vi "Gas-Control-GUI.vi"() -> ()   [LabVIEW 2021]
uses:
  Controls/AR-Auto-Fill.ctl
  Controls/AR-Auto-Purge.ctl
  Controls/AR-DO-Action.ctl
panel:
  out "Data":bool[](array[boolean])
  in  "1000T Sim 2":dbl=1.0
  in  ">750 sim 2":bool=TRUE
  in  "10T Sim 2":dbl=10.0
  in  "<0.1T sim 2":bool
  out "Purge State":T1
  in  "1000T Sim":dbl=1.0
  in  ">750 sim":bool=TRUE
  in  "<0.01T sim":bool
  in  "10T Sim":dbl=10.0
  in  "simulate":bool
  out "Fill State":T2
  out "O2 pwr":bool
  out "Gas SOL":bool
  out "Vac SOL":bool
  in  "Quit":bool
  out "Purge Done":bool
  in  "Auto purge":bool
  out "0-25% O2 (AI2)":dbl caption="0-25% O2" format="%.1f %"
  out "O2 1000ppm (AI3)":dbl caption="1000 PPM O2" format="%.0f PPM"
  out "1000 Torr (AI1)":dbl caption="1000 Torr Gage" format="%.1f Torr"
  out "10 Torr (AI0)":dbl caption="10 Torr Gage" format="%.2f Torr"
  out "Gage Err (DI2)":bool
  out "O2 Timer":dbl format="%.1f sec"
  in  "O2 1000ppm (DO3)":bool
  out "Gas sol timer":dbl caption="Gas Solenoid Timer" format="%.1f sec"
  in  "Gas sol (DO2)":bool
  in  "Vac sol (DO1)":bool
  out "Vac sol timer":dbl caption="Vac Solenoid Timer" format="%.1f sec"
  in  "Pump (DO0)":bool
  out "Fill Done":bool
  in  "Auto fill":bool
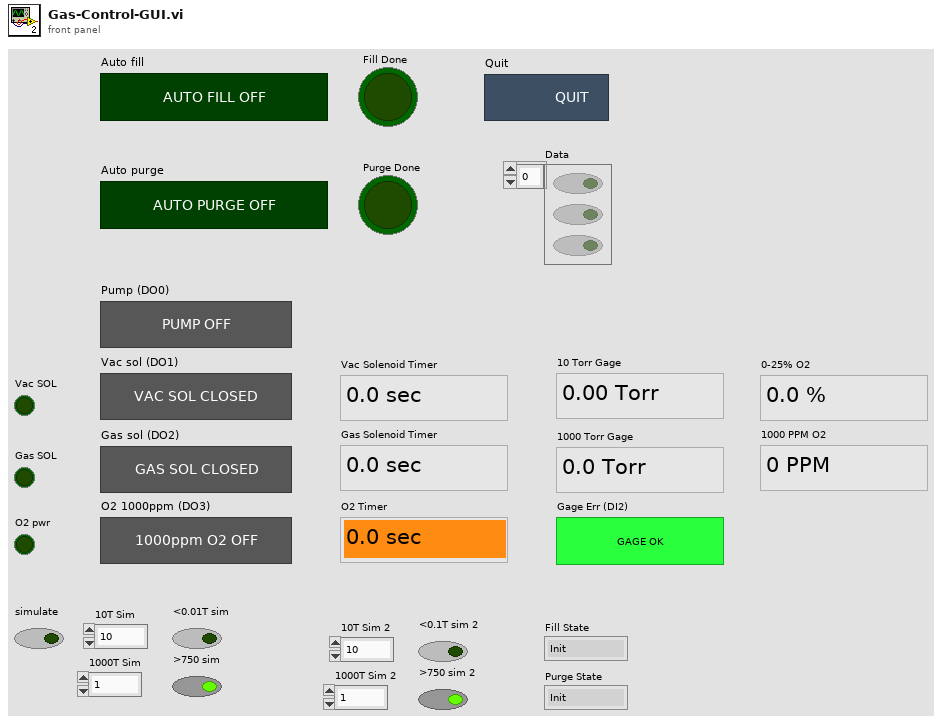
[diagram p1: front panel]
types:
  T1 = typedef "AR-Auto-Purge.ctl" = enum16{"Init", "Start Pump", "Stop Pump", "10T Gage", "1000T Gage", "End"}
  T2 = typedef "AR-Auto-Fill.ctl" = enum16{"Init", "Start Pump", "Stop Pump", "Gas Open", "Gas Close", "10T Gage", "1000T Gage", "End"}
  T3 = typedef "AR-DO-Action.ctl" = enum16{"Init", "Update", "Keep DO3"}
  T4 = enum8{"Enabled", "Disabled", "Disabled and Grayed Out"}
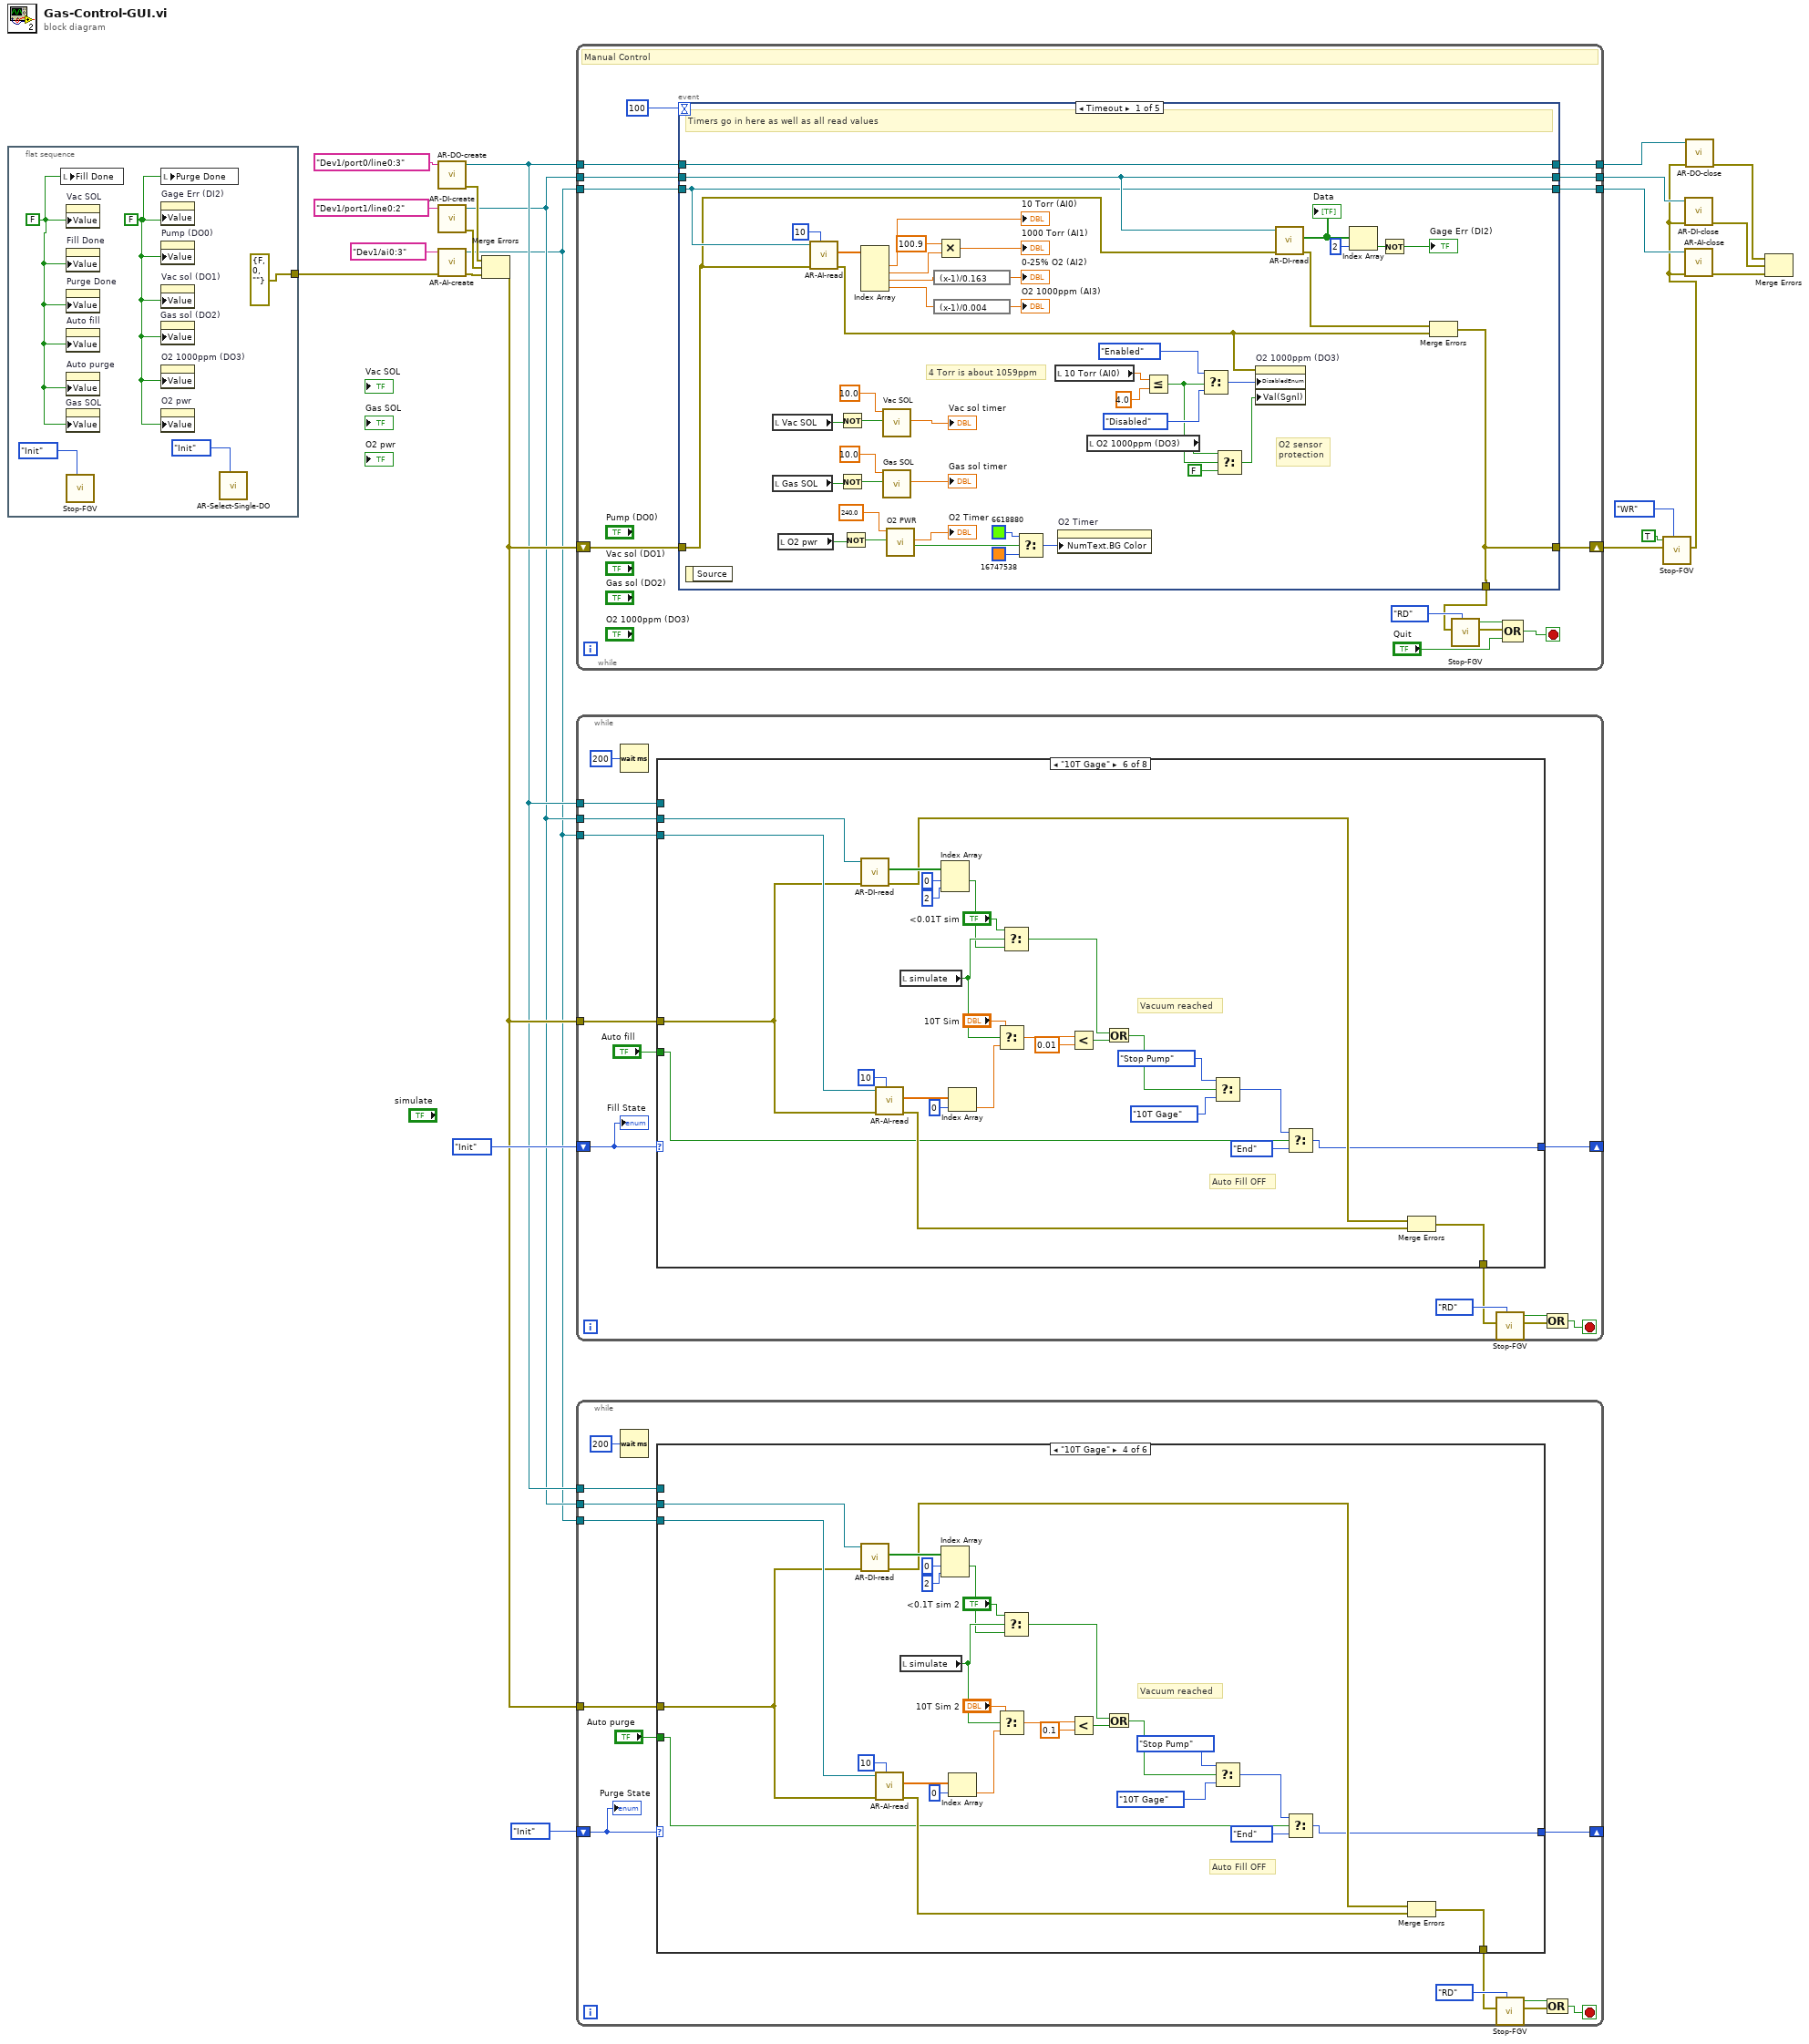
[diagram p0: block diagram]
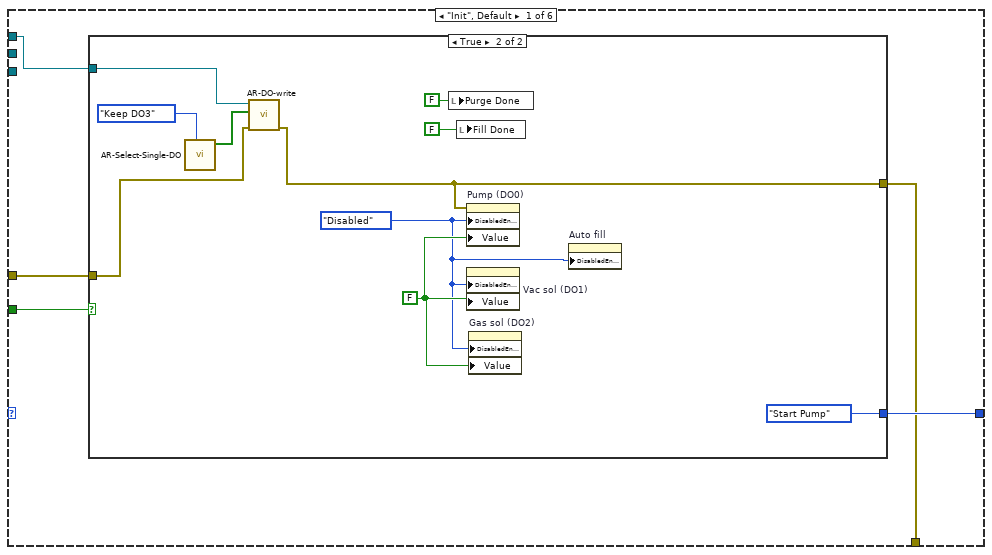
[diagram p2: hidden frame]
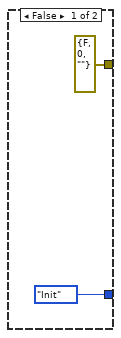
[diagram p3: hidden frame]
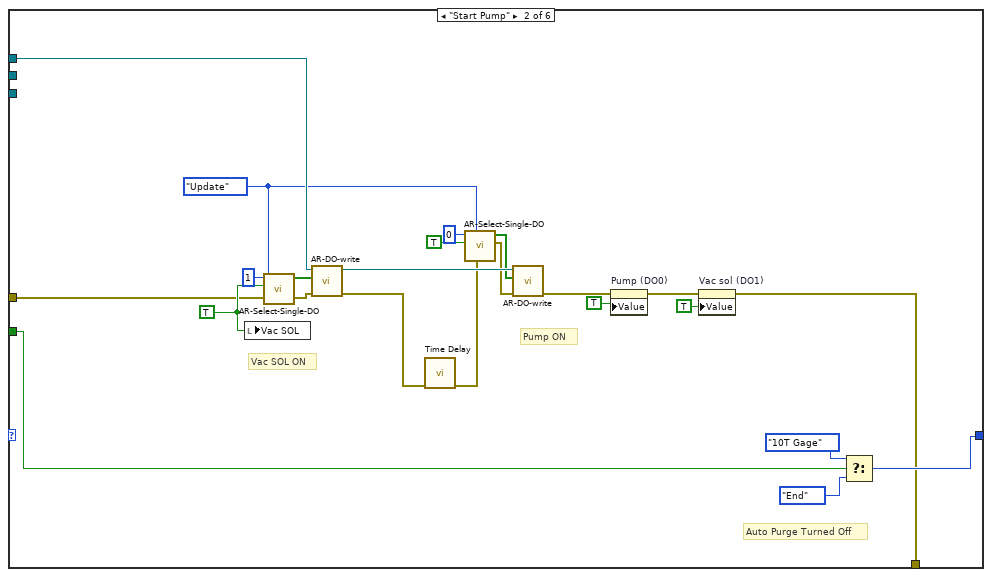
[diagram p4: hidden frame]
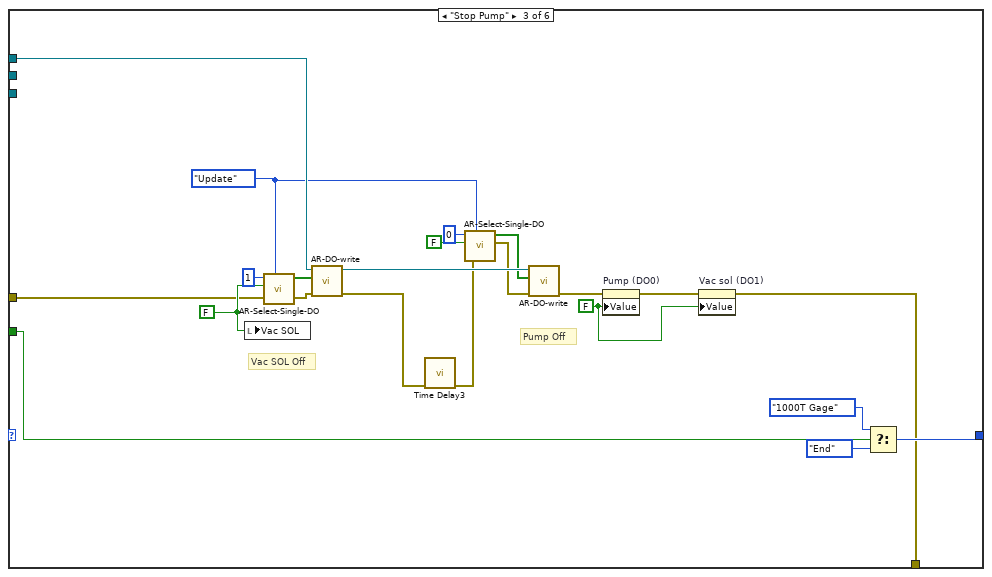
[diagram p5: hidden frame]
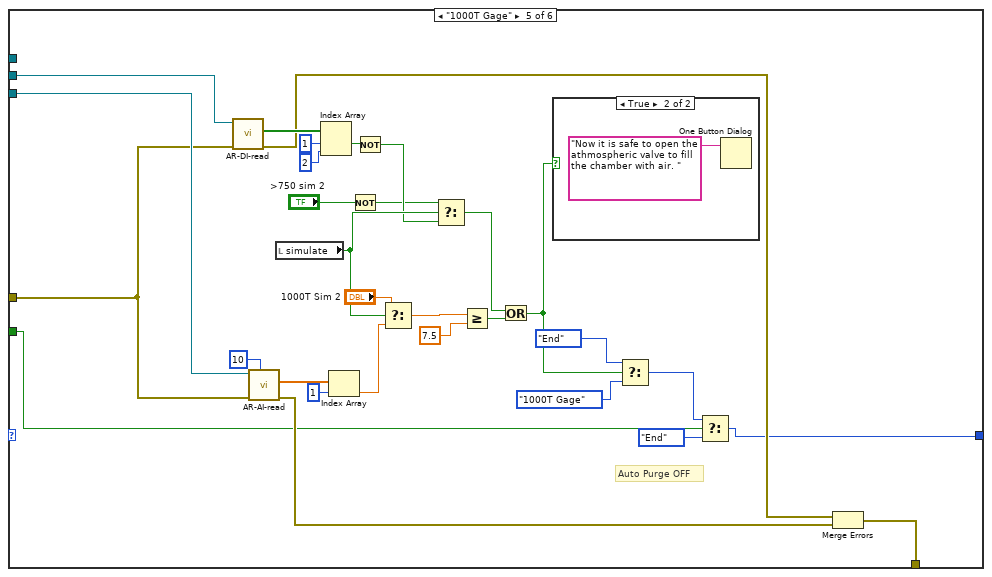
[diagram p6: hidden frame]
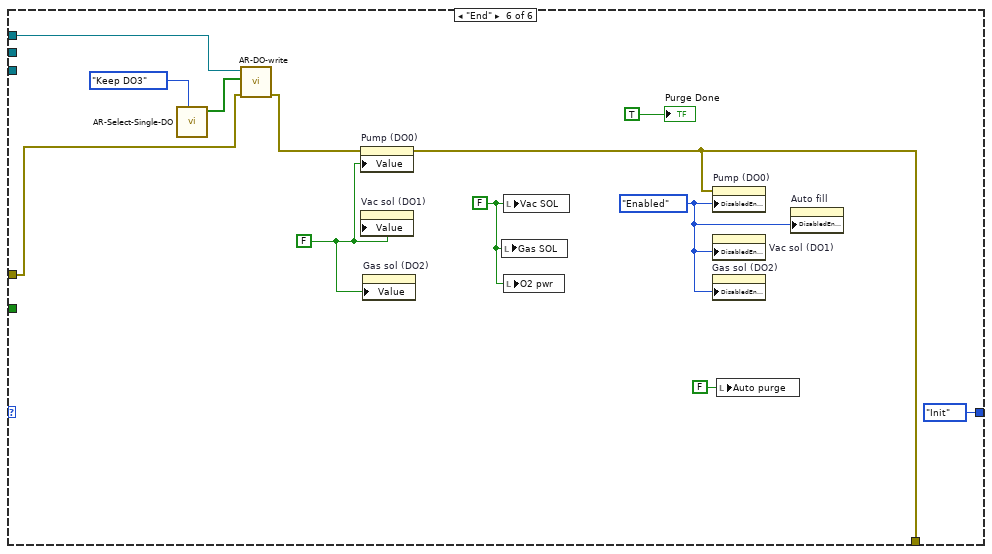
[diagram p8: hidden frame]
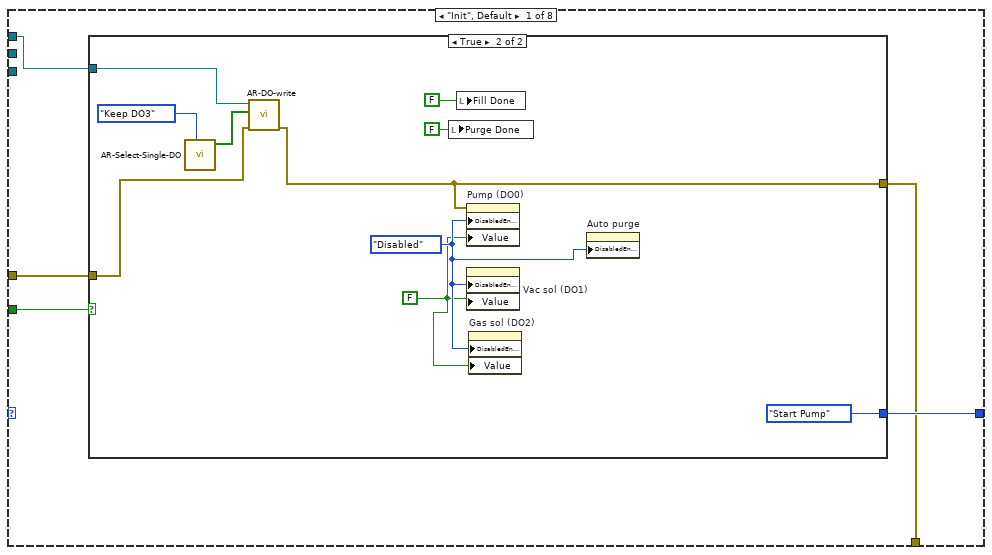
[diagram p9: hidden frame]
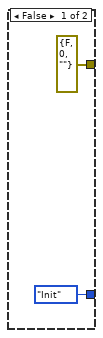
[diagram p10: hidden frame]
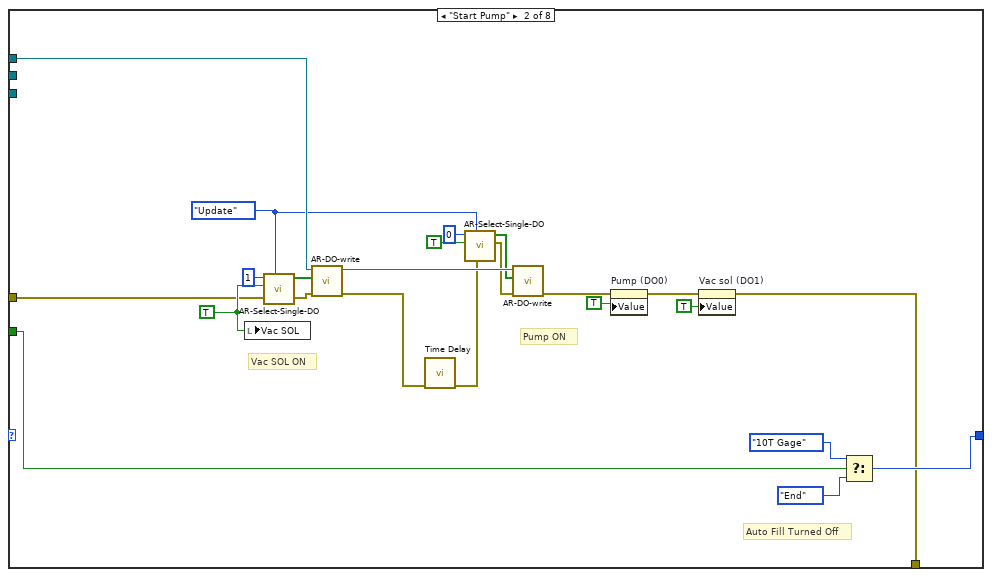
[diagram p11: hidden frame]
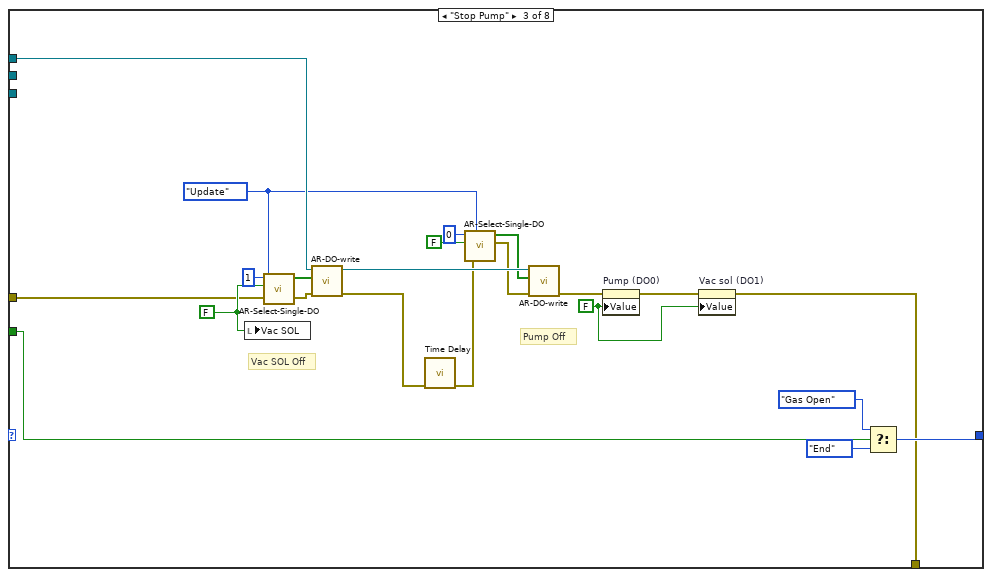
[diagram p12: hidden frame]
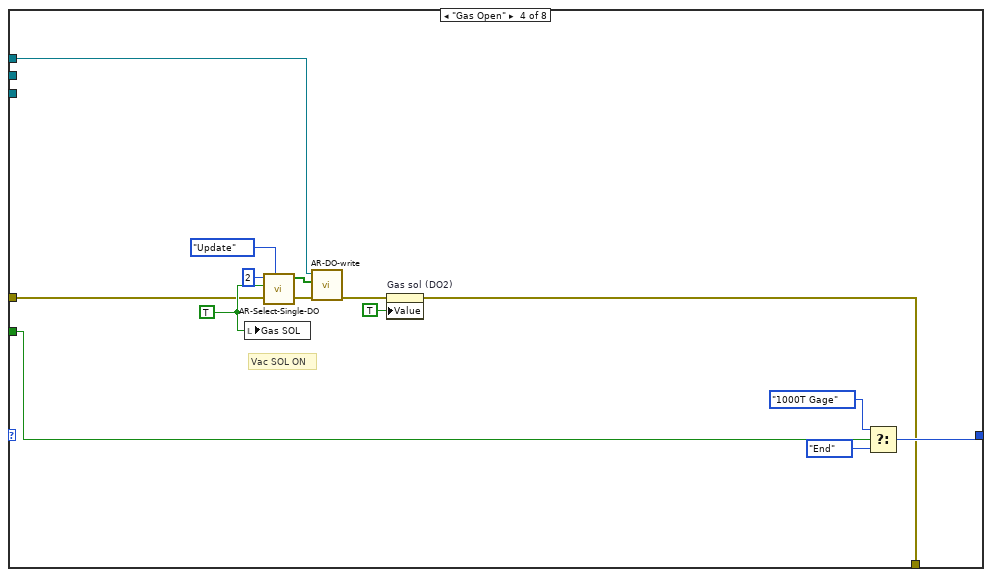
[diagram p13: hidden frame]
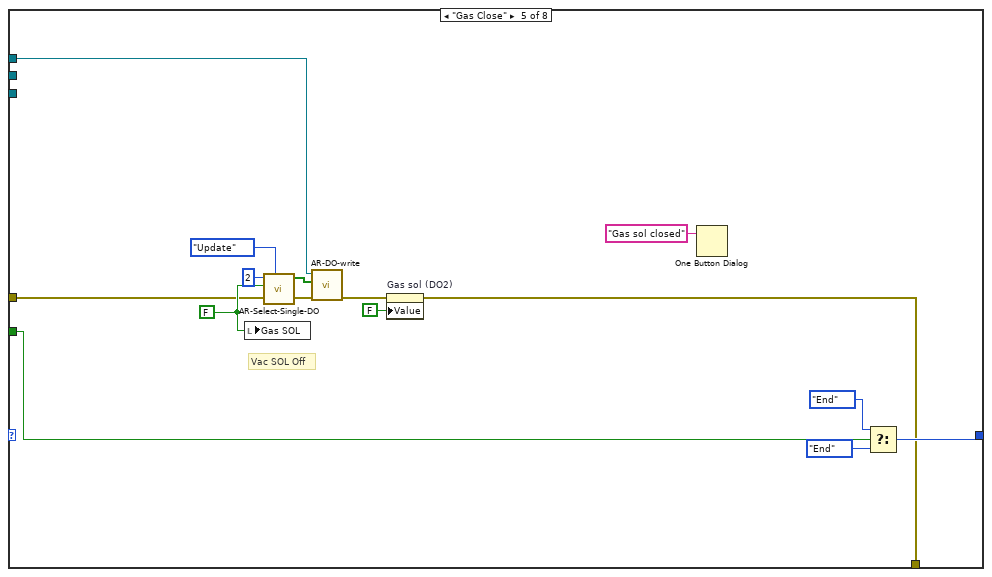
[diagram p14: hidden frame]
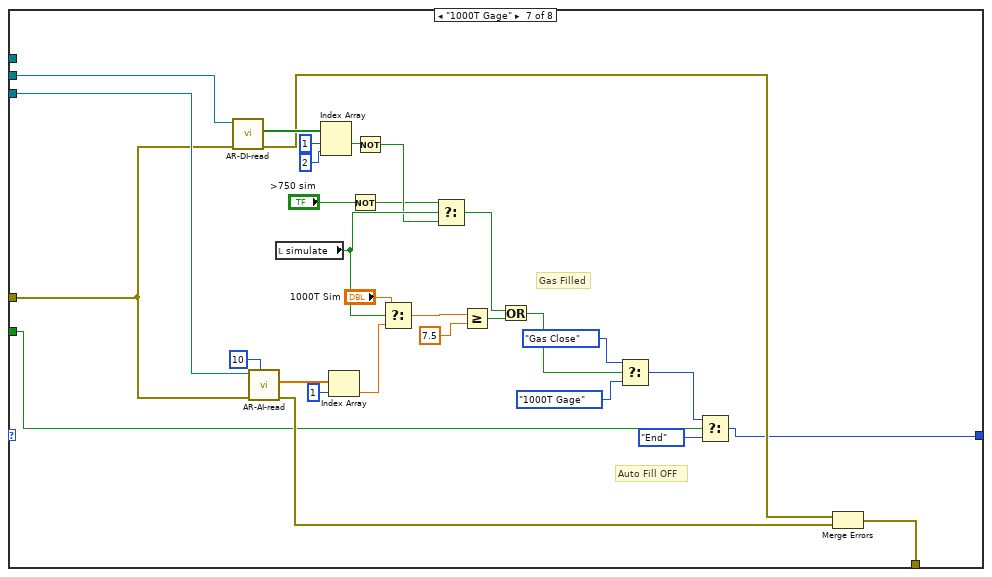
[diagram p15: hidden frame]
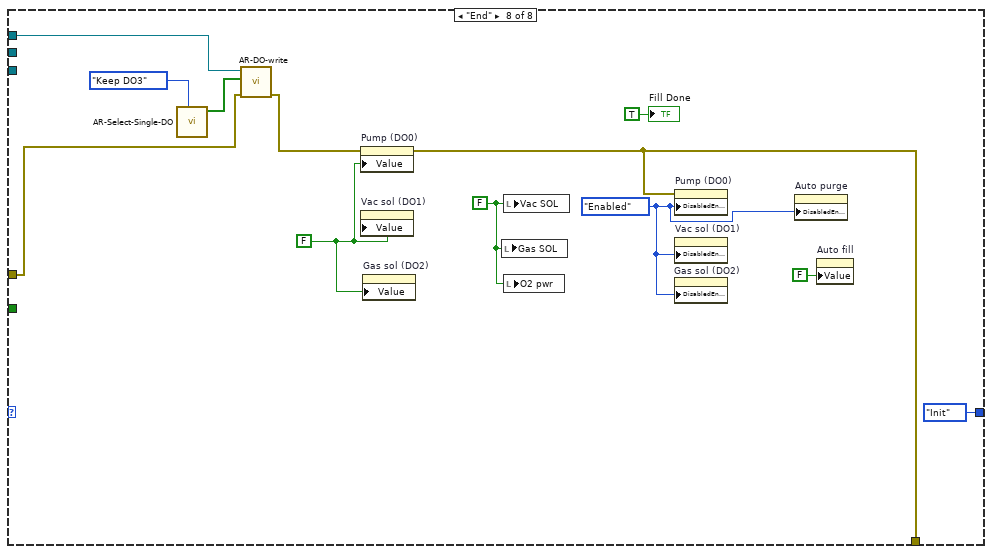
[diagram p16: hidden frame]
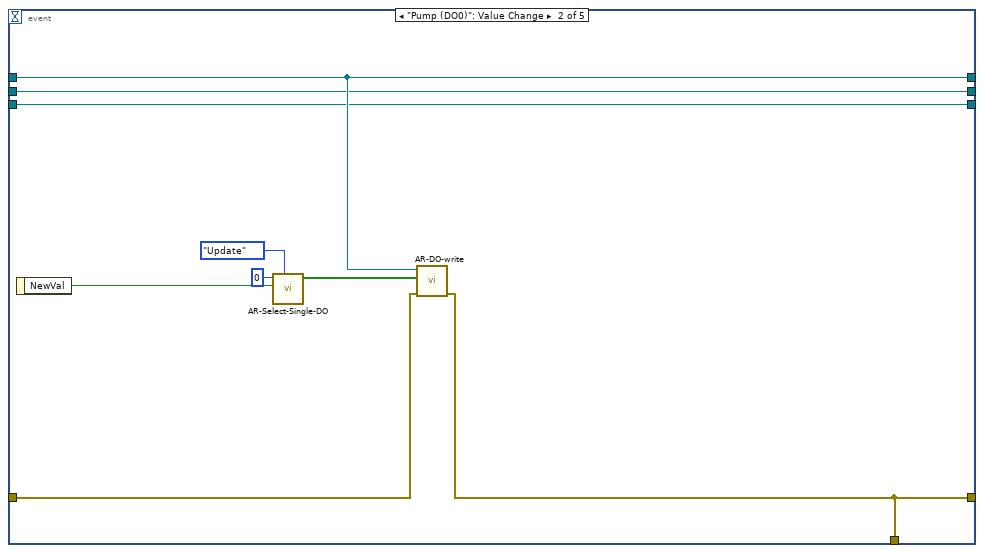
[diagram p17: hidden frame]
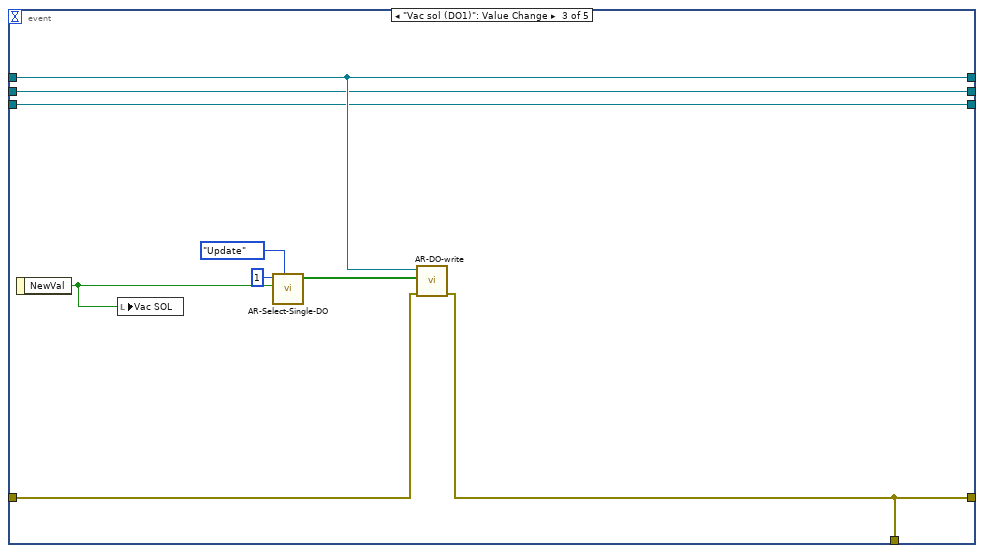
[diagram p18: hidden frame]
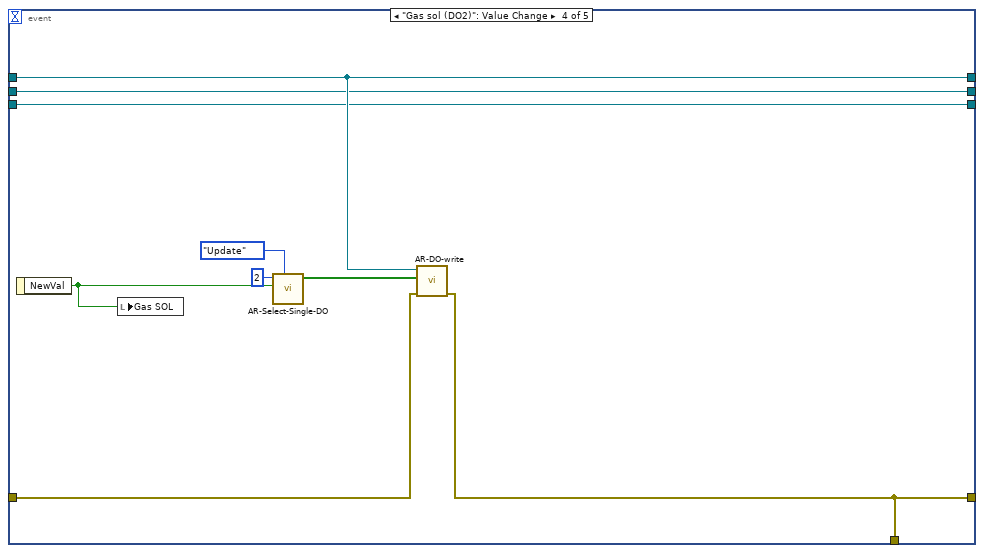
[diagram p19: hidden frame]
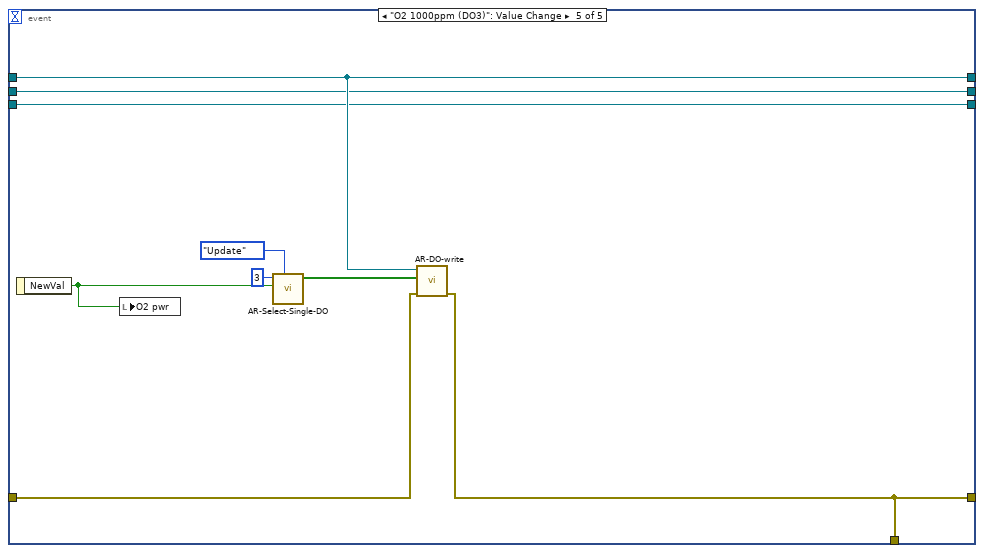
[diagram p20: hidden frame]
diagram:
  n1 = flat-sequence {
    tunnel: [errorcluster {"status"=FALSE, "code"=0, "source"=""} ("error out")] -> w11
    frame #0 {
      w25 = FALSE ("Vac SOL")
      w26 = FALSE ("Vac SOL")
      n2 = local write "Fill Done"(w26) -> ()
      n3 = property on="Vac SOL" class="Bool (strict)"("Value"=w26) -> ()  [unwired: 2 in, 2 out]
      n4 = property on="Fill Done" class="Bool (strict)"("Value"=w26) -> ()  [unwired: 2 in, 2 out]
      n5 = property on="Purge Done" class="Bool (strict)"("Value"=w26) -> ()  [unwired: 2 in, 2 out]
      n6 = property on="Auto fill" class="Bool (strict)"("Value"=w26) -> ()  [unwired: 2 in, 2 out]
      n7 = property on="Auto purge" class="Bool (strict)"("Value"=w26) -> ()  [unwired: 2 in, 2 out]
      n8 = property on="Gas SOL" class="Bool (strict)"("Value"=w26) -> ()  [unwired: 2 in, 2 out]
      n9 = call "Stop-FGV.vi"("Action (RD)"=enum16{"Init", "WR", "RD"}."Init") -> ()  [unwired: 9 in, 2 out]
      n10 = local write "Purge Done"(w25) -> ()
      n11 = property on="Gage Err (DI2)" class="Bool"("Value"=w25) -> ()  [unwired: 2 in, 2 out]
      n12 = property on="Pump (DO0)" class="Bool (strict)"("Value"=w25) -> ()  [unwired: 2 in, 2 out]
      n13 = property on="Vac sol (DO1)" class="Bool (strict)"("Value"=w25) -> ()  [unwired: 2 in, 2 out]
      n14 = property on="Gas sol (DO2)" class="Bool (strict)"("Value"=w25) -> ()  [unwired: 2 in, 2 out]
      n15 = property on="O2 1000ppm (DO3)" class="Bool (strict)"("Value"=w25) -> ()  [unwired: 2 in, 2 out]
      n16 = property on="O2 pwr" class="Bool (strict)"("Value"=w25) -> ()  [unwired: 2 in, 2 out]
      n17 = call "AR-Select-Single-DO.vi"("Action"=AR-DO-Action."Init") -> ()  [unwired: 9 in, 2 out]
    }
  }
  n18 = call "AR-DO-create.vi"("lines"=tag "Dev1/port0/line0:3") -> ("error out"=w14:errorcluster, "DO task out"=w4:refnum<k21>)  [unwired: 9 in]
  n19 = call "AR-DI-create.vi"("lines"=tag "Dev1/port1/line0:2") -> ("error out"=w13:errorcluster, "DI task out"=w3:refnum<k21>)  [unwired: 9 in]
  n20 = call "AR-AI-create.vi"("error in"=w11, "lines"=tag "Dev1/ai0:3") -> ("error out"=w12:errorcluster, "AI task out"=w2:refnum<k21>)  [unwired: 8 in]
  n21 = Merge Errors(w14, w13, w12) -> (w5:errorcluster)
  n22 = while {
    tunnel: w4 -> [w42]
    tunnel: w3 -> [w41]
    tunnel: w2 -> [w40]
    shift-right: [w39] -> w8
    shift-left: w5 -> [w38]
    tunnel: [w35] -> w20
    tunnel: [w34] -> w19
    tunnel: [w33] -> w18
    stop <- w37 stop-if-true
    # "Manual Control"
    n23 = event shown="[0] Timeout" {
      selector: _ -> [_ _ _ _ _]
      dyn-events: _ -> [_ _ _ _ _]
      timeout: 100 -> [_ _ _ _ _]
      tunnel: w42 -> [w80 w92 w102 w111 w120]
      tunnel: w41 -> [w79 w91 w101 w110 w119]
      tunnel: w40 -> [w78 w90 w100 w109 w118]
      tunnel: [w77 w93 w103 w112 w121] -> w39
      tunnel: w38 -> [w75 w94 w104 w113 w122]
      tunnel: [w77 w93 w103 w112 w121] -> w31
      tunnel: [w80 w92 w102 w111 w120] -> w35
      tunnel: [w79 w91 w101 w110 w119] -> w34
      tunnel: [w78 w90 w100 w109 w118] -> w33
      event Timeout {
        # "O2 sensor\nprotection"
        # "4 Torr is about 1059ppm"
        # "Timers go in here as well as all read values"
        n24 = event-data() -> ()  [unwired: 1 in, 1 out]
        n25 = local read "Vac SOL"() -> (w88:bool)
        n26 = local read "Gas SOL"() -> (w73:bool)
        n27 = local read "O2 pwr"() -> (w69:bool)
        n28 = call "AR-AI-read.vi"("number of samples"=10, "error in"=w75, "AI task in"=w78) -> ("error out"=w51:errorcluster, "Data"=w83:dbl[])  [unwired: 6 in, 1 out]
        n29 = Not(x=w88) -> (.not. x?=w89:bool)
        n30 = Not(x=w73) -> (.not. x?=w72:bool)
        n31 = Not(x=w69) -> (.not. x?=w70:bool)
        n32 = Index Array(array=w83) -> (element #1=→"10 Torr (AI0)":dbl, element #2=w62:dbl, element #3=w59:dbl, element #4=w56:dbl)  [unwired: 4 in]
        n33 = call "Vac SOL"("Time Target (s)"=10.0, "Reset"=w89) -> ("Elapsed Time (s)"=→"Vac sol timer":dbl)  [unwired: 10 in, 7 out]
        n34 = call "Gas SOL"("Time Target (s)"=10.0, "Reset"=w72) -> ("Elapsed Time (s)"=→"Gas sol timer":dbl)  [unwired: 10 in, 7 out]
        n35 = call "O2 PWR"("Time Target (s)"=240.0, "Reset"=w70) -> ("Elapsed Time (s)"=→"O2 Timer":dbl, "Time has Elapsed"=w65:bool)  [unwired: 10 in, 6 out]
        n36 = expression code="(x-1)/0.163"(w59) -> (→"0-25% O2 (AI2)":dbl)
        n37 = expression code="(x-1)/0.004"(w56) -> (→"O2 1000ppm (AI3)":dbl)
        n38 = Multiply(x=100.9, y=w62) -> (x*y=→"1000 Torr (AI1)":dbl)
        n39 = Select(t=u32 6618880 ("Numeric Text.Colors:BG Color"), s=w65, f=u32 16747538 ("Numeric Text.Colors:BG Color")) -> (s? t:f=w63:u32)
        n40 = local read "10 Torr (AI0)"() -> (w55:dbl)
        n41 = property on="O2 Timer" class="DigNum (strict)"("NumText.BG Color"=w63) -> ()  [unwired: 2 in, 2 out]
        n42 = local read "O2 1000ppm (DO3)"() -> (w48:bool)
        n43 = Less Or Equal?(x=w55, y=4.0) -> (x <= y?=w49:bool)
        n44 = Select(t=T4."Enabled" ("Disabled"), s=w49, f=T4."Disabled" ("Disabled")) -> (s? t:f=w50:T4)
        n45 = Select(t=w48, s=w49, f=FALSE) -> (s? t:f=w46:bool)
        n46 = property on="O2 1000ppm (DO3)" class="Bool (strict)"(error in=w51, "DisabledEnum"=w50, "Val(Sgnl)"=w46) -> ()  [unwired: 1 in, 2 out]
        n47 = call "AR-DI-read.vi"("error in"=w75, "DI task in"=w79) -> ("error out"=w81:errorcluster, "Data"=w86:bool[])  [unwired: 7 in, 1 out]
        "Data" <- w86
        n48 = Index Array(array=w86, index=2) -> (element=w45:bool)
        n49 = Not(x=w45) -> (.not. x?=→"Gage Err (DI2)":bool)
        n50 = Merge Errors(w81, w51) -> (w77:errorcluster)
      }
      event "Pump (DO0)": Value Change {
        n51 = event-data() -> ("NewVal"=w95:bool)  [unwired: 1 in]
        n52 = call "AR-Select-Single-DO.vi"("Action"=enum16{"Init", "Update"}."Update", "DO"=w95, "index"=0) -> ("DO Data"=w97:bool[])  [unwired: 7 in, 1 out]
        n53 = call "AR-DO-write.vi"("error in (no error)"=w94, "Data"=w97, "DO task in"=w92) -> ("error out"=w93:errorcluster)  [unwired: 7 in, 1 out]
      }
      event "Vac sol (DO1)": Value Change {
        n54 = event-data() -> ("NewVal"=w99:bool)  [unwired: 1 in]
        n55 = local write "Vac SOL"(w99) -> ()
        n56 = call "AR-Select-Single-DO.vi"("Action"=enum16{"Init", "Update"}."Update", "DO"=w99, "index"=1) -> ("DO Data"=w106:bool[])  [unwired: 7 in, 1 out]
        n57 = call "AR-DO-write.vi"("error in (no error)"=w104, "Data"=w106, "DO task in"=w102) -> ("error out"=w103:errorcluster)  [unwired: 7 in, 1 out]
      }
      event "Gas sol (DO2)": Value Change {
        n58 = event-data() -> ("NewVal"=w108:bool)  [unwired: 1 in]
        n59 = local write "Gas SOL"(w108) -> ()
        n60 = call "AR-Select-Single-DO.vi"("Action"=enum16{"Init", "Update"}."Update", "DO"=w108, "index"=2) -> ("DO Data"=w115:bool[])  [unwired: 7 in, 1 out]
        n61 = call "AR-DO-write.vi"("error in (no error)"=w113, "Data"=w115, "DO task in"=w111) -> ("error out"=w112:errorcluster)  [unwired: 7 in, 1 out]
      }
      event "O2 1000ppm (DO3)": Value Change {
        n62 = event-data() -> ("NewVal"=w117:bool)  [unwired: 1 in]
        n63 = local write "O2 pwr"(w117) -> ()
        n64 = call "AR-Select-Single-DO.vi"("Action"=enum16{"Init", "Update"}."Update", "DO"=w117, "index"=3) -> ("DO Data"=w124:bool[])  [unwired: 7 in, 1 out]
        n65 = call "AR-DO-write.vi"("error in (no error)"=w122, "Data"=w124, "DO task in"=w120) -> ("error out"=w121:errorcluster)  [unwired: 7 in, 1 out]
      }
    }
    n66 = call "Stop-FGV.vi"("Action (RD)"=enum16{"Init", "WR", "RD"}."RD", "error in"=w31) -> ("error out"=w30:errorcluster, "Out"=w29:bool)  [unwired: 8 in]
    n67 = Compound Arithmetic op=OR(w29, w30, "Quit") -> (w37:bool)
  }
  n68 = while {
    tunnel: w4 -> [w130]
    tunnel: w3 -> [w126]
    tunnel: w2 -> [w127]
    shift-right: [w132] -> _
    shift-left: AR-Auto-Fill."Init" ("Fill State") -> [w131]
    tunnel: w5 -> [w128]
    stop <- w135 stop-if-true
    n69 = Wait (ms)(milliseconds to wait=u32 200) -> ()  [unwired: 1 out]
    n70 = case shown="\"10T Gage\"" w131 {
      tunnel: "Auto fill" -> [w143 w167 w188 w206 w220 w230 w262 _]
      tunnel: [w142 w164 w185 w203 w217 w227 w259 AR-Auto-Fill."Init" ("f")] -> w132
      tunnel: w130 -> [w141 w175 w196 w209 w223 _ _ w292]
      tunnel: [w140 w159 w181 w201 w215 w231 w263 w285] -> w129
      tunnel: w128 -> [w139 w168 w189 w207 w221 w244 w274 w291]
      tunnel: w127 -> [_ _ _ _ _ w252 w282 _]
      tunnel: w126 -> [_ _ _ _ _ w245 w275 _]
      frame "Init", Default {
        n71 = case shown="True" w143 {
          tunnel: [AR-Auto-Fill."Init" ("Fill State") AR-Auto-Fill."Start Pump" ("Fill State")] -> w142
          tunnel: w141 -> [_ w153]
          tunnel: [errorcluster {"status"=FALSE, "code"=0, "source"=""} ("error out") w149] -> w140
          tunnel: w139 -> [_ w151]
          frame False {
          }
          frame True {
            w150 = FALSE
            w155 = T4."Disabled" ("Disabled")
            n72 = call "AR-Select-Single-DO.vi"("Action"=AR-DO-Action."Keep DO3") -> ("DO Data"=w152:bool[])  [unwired: 9 in, 1 out]
            n73 = call "AR-DO-write.vi"("error in (no error)"=w151, "Data"=w152, "DO task in"=w153) -> ("error out"=w149:errorcluster)  [unwired: 7 in, 1 out]
            n74 = local write "Purge Done"(FALSE ("Purge Done")) -> ()
            n75 = local write "Fill Done"(FALSE ("Purge Done")) -> ()
            n76 = property on="Pump (DO0)" class="Bool (strict)"(error in=w149, "DisabledEnum"=w155, "Value"=w150) -> ()  [unwired: 1 in, 2 out]
            n77 = property on="Vac sol (DO1)" class="Bool (strict)"("DisabledEnum"=w155, "Value"=w150) -> ()  [unwired: 2 in, 2 out]
            n78 = property on="Gas sol (DO2)" class="Bool (strict)"("DisabledEnum"=w155, "Value"=w150) -> ()  [unwired: 2 in, 2 out]
            n79 = property on="Auto purge" class="Bool (strict)"("DisabledEnum"=w155) -> ()  [unwired: 2 in, 2 out]
          }
        }
      }
      frame "Start Pump" {
        w156 = AR-DO-Action."Update" ("Action")
        w174 = TRUE ("DO")
        # "Auto Fill Turned Off"
        # "Pump ON"
        # "Vac SOL ON"
        n80 = local write "Vac SOL"(w174) -> ()
        n81 = call "AR-Select-Single-DO.vi"("Action"=w156, "DO"=w174, "index"=1) -> ("DO Data"=w176:bool[])  [unwired: 7 in, 1 out]
        n82 = call "AR-DO-write.vi"("error in (no error)"=w168, "Data"=w176, "DO task in"=w175) -> ("error out"=w169:errorcluster, "DO task out"=w172:refnum<k21>)  [unwired: 7 in]
        n83 = call "Time Delay"("error in (no error)"=w169) -> ("error out"=w158:errorcluster)  [unwired: 10 in]
        n84 = call "AR-Select-Single-DO.vi"("error in (no error)"=w158, "Action"=w156, "DO"=TRUE, "index"=0) -> ("error out"=w157:errorcluster, "DO Data"=w171:bool[])  [unwired: 6 in]
        n85 = call "AR-DO-write.vi"("error in (no error)"=w157, "Data"=w171, "DO task in"=w172) -> ("error out"=w162:errorcluster)  [unwired: 7 in, 1 out]
        n86 = property on="Pump (DO0)" class="Bool (strict)"(error in=w162, "Value"=TRUE ("Pump (DO0)")) -> (error out=w161:errorcluster)  [unwired: 1 in, 1 out]
        n87 = property on="Vac sol (DO1)" class="Bool (strict)"(error in=w161, "Value"=TRUE ("Vac sol (DO1)")) -> (error out=w159:errorcluster)  [unwired: 1 in, 1 out]
        n88 = Select(t=AR-Auto-Fill."10T Gage" ("Fill State"), s=w167, f=AR-Auto-Fill."End" ("Fill State")) -> (s? t:f=w164:T2)
      }
      frame "Stop Pump" {
        w178 = AR-DO-Action."Update" ("Action")
        w182 = FALSE ("Pump (DO0)")
        w195 = FALSE ("DO")
        # "Pump Off"
        # "Vac SOL Off"
        n89 = local write "Vac SOL"(w195) -> ()
        n90 = call "AR-Select-Single-DO.vi"("Action"=w178, "DO"=w195, "index"=1) -> ("DO Data"=w197:bool[])  [unwired: 7 in, 1 out]
        n91 = call "AR-DO-write.vi"("error in (no error)"=w189, "Data"=w197, "DO task in"=w196) -> ("error out"=w190:errorcluster, "DO task out"=w193:refnum<k21>)  [unwired: 7 in]
        n92 = call "Time Delay"("error in (no error)"=w190) -> ("error out"=w180:errorcluster)  [unwired: 10 in]
        n93 = call "AR-Select-Single-DO.vi"("error in (no error)"=w180, "Action"=w178, "DO"=FALSE, "index"=0) -> ("error out"=w179:errorcluster, "DO Data"=w192:bool[])  [unwired: 6 in]
        n94 = call "AR-DO-write.vi"("error in (no error)"=w179, "Data"=w192, "DO task in"=w193) -> ("error out"=w184:errorcluster)  [unwired: 7 in, 1 out]
        n95 = property on="Pump (DO0)" class="Bool (strict)"(error in=w184, "Value"=w182) -> (error out=w183:errorcluster)  [unwired: 1 in, 1 out]
        n96 = property on="Vac sol (DO1)" class="Bool (strict)"(error in=w183, "Value"=w182) -> (error out=w181:errorcluster)  [unwired: 1 in, 1 out]
        n97 = Select(t=AR-Auto-Fill."Gas Open" ("Fill State"), s=w188, f=AR-Auto-Fill."End") -> (s? t:f=w185:T2)
      }
      frame "Gas Open" {
        w208 = TRUE ("DO")
        # "Vac SOL ON"
        n98 = local write "Gas SOL"(w208) -> ()
        n99 = call "AR-Select-Single-DO.vi"("Action"=AR-DO-Action."Update", "DO"=w208, "index"=2) -> ("DO Data"=w210:bool[])  [unwired: 7 in, 1 out]
        n100 = call "AR-DO-write.vi"("error in (no error)"=w207, "Data"=w210, "DO task in"=w209) -> ("error out"=w202:errorcluster)  [unwired: 7 in, 1 out]
        n101 = property on="Gas sol (DO2)" class="Bool (strict)"(error in=w202, "Value"=TRUE ("Gas sol (DO2)")) -> (error out=w201:errorcluster)  [unwired: 1 in, 1 out]
        n102 = Select(t=AR-Auto-Fill."1000T Gage" ("Fill State"), s=w206, f=AR-Auto-Fill."End") -> (s? t:f=w203:T2)
      }
      frame "Gas Close" {
        w222 = FALSE ("DO")
        # "Vac SOL Off"
        n103 = local write "Gas SOL"(w222) -> ()
        n104 = call "AR-Select-Single-DO.vi"("Action"=AR-DO-Action."Update", "DO"=w222, "index"=2) -> ("DO Data"=w224:bool[])  [unwired: 7 in, 1 out]
        n105 = call "AR-DO-write.vi"("error in (no error)"=w221, "Data"=w224, "DO task in"=w223) -> ("error out"=w216:errorcluster)  [unwired: 7 in, 1 out]
        n106 = property on="Gas sol (DO2)" class="Bool (strict)"(error in=w216, "Value"=FALSE ("Gas sol (DO2)")) -> (error out=w215:errorcluster)  [unwired: 1 in, 1 out]
        n107 = One Button Dialog(message="Gas sol closed") -> ()  [unwired: 1 in, 1 out]
        n108 = Select(t=AR-Auto-Fill."End" ("Fill State"), s=w220, f=AR-Auto-Fill."End") -> (s? t:f=w217:T2)
      }
      frame "10T Gage" {
        # "Auto Fill OFF"
        # "Vacuum reached"
        n109 = call "AR-DI-read.vi"("error in"=w244, "DI task in"=w245) -> ("error out"=w232:errorcluster, "Data"=w243:bool[])  [unwired: 7 in, 1 out]
        n110 = call "AR-AI-read.vi"("number of samples"=10, "error in"=w244, "AI task in"=w252) -> ("error out"=w233:errorcluster, "Data"=w251:dbl[])  [unwired: 6 in, 1 out]
        n111 = local read "simulate"() -> (w240:bool)
        n112 = Index Array(array=w243, index #1=0 ("index"), index #2=2 ("index")) -> (element #1=w239:bool)  [unwired: 1 out]
        n113 = Index Array(array=w251, index=0) -> (element=w249:dbl)
        n114 = Select(t="10T Sim", s=w240, f=w249) -> (s? t:f=w247:dbl)
        n115 = Select(t="<0.01T sim", s=w240, f=w239) -> (s? t:f=w237:bool)
        n116 = Less?(x=w247, y=0.01) -> (x < y?=w226:bool)
        n117 = Or(x=w237, y=w226) -> (x .or. y?=w236:bool)
        n118 = Select(t=AR-Auto-Fill."Stop Pump" ("Fill State"), s=w236, f=AR-Auto-Fill."10T Gage") -> (s? t:f=w229:T2)
        n119 = Select(t=w229, s=w230, f=AR-Auto-Fill."End") -> (s? t:f=w227:T2)
        n120 = Merge Errors(w232, w233) -> (w231:errorcluster)
      }
      frame "1000T Gage" {
        # "Auto Fill OFF"
        # "Gas Filled"
        n121 = call "AR-DI-read.vi"("error in"=w274, "DI task in"=w275) -> ("error out"=w264:errorcluster, "Data"=w273:bool[])  [unwired: 7 in, 1 out]
        n122 = call "AR-AI-read.vi"("number of samples"=10, "error in"=w274, "AI task in"=w282) -> ("error out"=w265:errorcluster, "Data"=w281:dbl[])  [unwired: 6 in, 1 out]
        n123 = local read "simulate"() -> (w270:bool)
        n124 = Index Array(array=w273, index #1=1 ("index"), index #2=2 ("index")) -> (element #1=w258:bool)  [unwired: 1 out]
        n125 = Index Array(array=w281, index=1) -> (element=w279:dbl)
        n126 = Not(x=">750 sim") -> (.not. x?=w255:bool)
        n127 = Not(x=w258) -> (.not. x?=w257:bool)
        n128 = Select(t="1000T Sim", s=w270, f=w279) -> (s? t:f=w277:dbl)
        n129 = Select(t=w255, s=w270, f=w257) -> (s? t:f=w269:bool)
        n130 = Greater Or Equal?(x=w277, y=7.5) -> (x >= y?=w254:bool)
        n131 = Or(x=w269, y=w254) -> (x .or. y?=w268:bool)
        n132 = Select(t=AR-Auto-Fill."Gas Close" ("Fill State"), s=w268, f=AR-Auto-Fill."1000T Gage") -> (s? t:f=w261:T2)
        n133 = Select(t=w261, s=w262, f=AR-Auto-Fill."End") -> (s? t:f=w259:T2)
        n134 = Merge Errors(w264, w265) -> (w263:errorcluster)
      }
      frame "End" {
        w286 = T4."Enabled" ("Disabled")
        w288 = FALSE ("Vac SOL")
        w289 = FALSE
        n135 = call "AR-Select-Single-DO.vi"("Action"=AR-DO-Action."Keep DO3") -> ("DO Data"=w293:bool[])  [unwired: 9 in, 1 out]
        n136 = call "AR-DO-write.vi"("error in (no error)"=w291, "Data"=w293, "DO task in"=w292) -> ("error out"=w290:errorcluster)  [unwired: 7 in, 1 out]
        n137 = property on="Pump (DO0)" class="Bool (strict)"(error in=w290, "Value"=w289) -> (error out=w285:errorcluster)  [unwired: 1 in, 1 out]
        n138 = property on="Vac sol (DO1)" class="Bool (strict)"("Value"=w289) -> ()  [unwired: 2 in, 2 out]
        n139 = property on="Gas sol (DO2)" class="Bool (strict)"("Value"=w289) -> ()  [unwired: 2 in, 2 out]
        n140 = local write "Gas SOL"(w288) -> ()
        n141 = local write "Vac SOL"(w288) -> ()
        n142 = local write "O2 pwr"(w288) -> ()
        n143 = property on="Pump (DO0)" class="Bool (strict)"(error in=w285, "DisabledEnum"=w286) -> ()  [unwired: 1 in, 2 out]
        n144 = property on="Vac sol (DO1)" class="Bool (strict)"("DisabledEnum"=w286) -> ()  [unwired: 2 in, 2 out]
        n145 = property on="Gas sol (DO2)" class="Bool (strict)"("DisabledEnum"=w286) -> ()  [unwired: 2 in, 2 out]
        n146 = property on="Auto purge" class="Bool (strict)"("DisabledEnum"=w286) -> ()  [unwired: 2 in, 2 out]
        n147 = property on="Auto fill" class="Bool (strict)"("Value"=FALSE ("Auto fill")) -> ()  [unwired: 2 in, 2 out]
        "Fill Done" <- TRUE ("Fill Done")
      }
    }
    n148 = call "Stop-FGV.vi"("Action (RD)"=enum16{"Init", "WR", "RD"}."RD", "error in"=w129) -> ("error out"=w137:errorcluster, "Out"=w138:bool)  [unwired: 8 in]
    n149 = Compound Arithmetic op=OR(w138, w137) -> (w135:bool)
    "Fill State" <- w131
  }
  n150 = while {
    tunnel: w4 -> [w301]
    tunnel: w3 -> [w297]
    tunnel: w2 -> [w298]
    shift-right: [w303] -> _
    shift-left: AR-Auto-Purge."Init" ("Purge State") -> [w302]
    tunnel: w5 -> [w299]
    stop <- w305 stop-if-true
    n151 = Wait (ms)(milliseconds to wait=u32 200) -> ()  [unwired: 1 out]
    n152 = case shown="\"10T Gage\"" w302 {
      tunnel: "Auto purge" -> [w313 w337 w358 w373 w406 _]
      tunnel: [w312 w334 w355 w370 w403 AR-Auto-Purge."Init" ("f")] -> w303
      tunnel: w301 -> [w311 w345 w366 _ _ w437]
      tunnel: [w310 w329 w351 w374 w407 w430] -> w300
      tunnel: w299 -> [w309 w338 w359 w387 w417 w436]
      tunnel: w298 -> [_ _ _ w395 w425 _]
      tunnel: w297 -> [_ _ _ w388 w418 _]
      frame "Init", Default {
        n153 = case shown="True" w313 {
          tunnel: [AR-Auto-Purge."Init" ("Purge State") AR-Auto-Purge."Start Pump" ("Fill State")] -> w312
          tunnel: w311 -> [_ w324]
          tunnel: [errorcluster {"status"=FALSE, "code"=0, "source"=""} ("error out") w320] -> w310
          tunnel: w309 -> [_ w322]
          frame False {
          }
          frame True {
            w321 = FALSE
            w318 = T4."Disabled" ("Disabled")
            n154 = call "AR-Select-Single-DO.vi"("Action"=AR-DO-Action."Keep DO3") -> ("DO Data"=w323:bool[])  [unwired: 9 in, 1 out]
            n155 = call "AR-DO-write.vi"("error in (no error)"=w322, "Data"=w323, "DO task in"=w324) -> ("error out"=w320:errorcluster)  [unwired: 7 in, 1 out]
            n156 = local write "Purge Done"(FALSE ("Purge Done")) -> ()
            n157 = local write "Fill Done"(FALSE ("Purge Done")) -> ()
            n158 = property on="Pump (DO0)" class="Bool (strict)"(error in=w320, "DisabledEnum"=w318, "Value"=w321) -> ()  [unwired: 1 in, 2 out]
            n159 = property on="Vac sol (DO1)" class="Bool (strict)"("DisabledEnum"=w318, "Value"=w321) -> ()  [unwired: 2 in, 2 out]
            n160 = property on="Gas sol (DO2)" class="Bool (strict)"("DisabledEnum"=w318, "Value"=w321) -> ()  [unwired: 2 in, 2 out]
            n161 = property on="Auto fill" class="Bool (strict)"("DisabledEnum"=w318) -> ()  [unwired: 2 in, 2 out]
          }
        }
      }
      frame "Start Pump" {
        w326 = AR-DO-Action."Update" ("Action")
        w344 = TRUE ("DO")
        # "Auto Purge Turned Off"
        # "Pump ON"
        # "Vac SOL ON"
        n162 = local write "Vac SOL"(w344) -> ()
        n163 = call "AR-Select-Single-DO.vi"("Action"=w326, "DO"=w344, "index"=1) -> ("DO Data"=w346:bool[])  [unwired: 7 in, 1 out]
        n164 = call "AR-DO-write.vi"("error in (no error)"=w338, "Data"=w346, "DO task in"=w345) -> ("error out"=w339:errorcluster, "DO task out"=w342:refnum<k21>)  [unwired: 7 in]
        n165 = call "Time Delay"("error in (no error)"=w339) -> ("error out"=w328:errorcluster)  [unwired: 10 in]
        n166 = call "AR-Select-Single-DO.vi"("error in (no error)"=w328, "Action"=w326, "DO"=TRUE, "index"=0) -> ("error out"=w327:errorcluster, "DO Data"=w341:bool[])  [unwired: 6 in]
        n167 = call "AR-DO-write.vi"("error in (no error)"=w327, "Data"=w341, "DO task in"=w342) -> ("error out"=w332:errorcluster)  [unwired: 7 in, 1 out]
        n168 = property on="Pump (DO0)" class="Bool (strict)"(error in=w332, "Value"=TRUE ("Pump (DO0)")) -> (error out=w331:errorcluster)  [unwired: 1 in, 1 out]
        n169 = property on="Vac sol (DO1)" class="Bool (strict)"(error in=w331, "Value"=TRUE ("Vac sol (DO1)")) -> (error out=w329:errorcluster)  [unwired: 1 in, 1 out]
        n170 = Select(t=AR-Auto-Purge."10T Gage" ("Purge State"), s=w337, f=AR-Auto-Purge."End" ("Purge State")) -> (s? t:f=w334:T1)
      }
      frame "Stop Pump" {
        w348 = AR-DO-Action."Update" ("Action")
        w352 = FALSE ("Pump (DO0)")
        w365 = FALSE ("DO")
        # "Pump Off"
        # "Vac SOL Off"
        n171 = local write "Vac SOL"(w365) -> ()
        n172 = call "AR-Select-Single-DO.vi"("Action"=w348, "DO"=w365, "index"=1) -> ("DO Data"=w367:bool[])  [unwired: 7 in, 1 out]
        n173 = call "AR-DO-write.vi"("error in (no error)"=w359, "Data"=w367, "DO task in"=w366) -> ("error out"=w360:errorcluster, "DO task out"=w363:refnum<k21>)  [unwired: 7 in]
        n174 = call "Time Delay3"("error in (no error)"=w360) -> ("error out"=w350:errorcluster)  [unwired: 10 in]
        n175 = call "AR-Select-Single-DO.vi"("error in (no error)"=w350, "Action"=w348, "DO"=FALSE, "index"=0) -> ("error out"=w349:errorcluster, "DO Data"=w362:bool[])  [unwired: 6 in]
        n176 = call "AR-DO-write.vi"("error in (no error)"=w349, "Data"=w362, "DO task in"=w363) -> ("error out"=w354:errorcluster)  [unwired: 7 in, 1 out]
        n177 = property on="Pump (DO0)" class="Bool (strict)"(error in=w354, "Value"=w352) -> (error out=w353:errorcluster)  [unwired: 1 in, 1 out]
        n178 = property on="Vac sol (DO1)" class="Bool (strict)"(error in=w353, "Value"=w352) -> (error out=w351:errorcluster)  [unwired: 1 in, 1 out]
        n179 = Select(t=AR-Auto-Purge."1000T Gage" ("Purge State"), s=w358, f=AR-Auto-Purge."End") -> (s? t:f=w355:T1)
      }
      frame "10T Gage" {
        # "Auto Fill OFF"
        # "Vacuum reached"
        n180 = call "AR-DI-read.vi"("error in"=w387, "DI task in"=w388) -> ("error out"=w375:errorcluster, "Data"=w386:bool[])  [unwired: 7 in, 1 out]
        n181 = call "AR-AI-read.vi"("number of samples"=10, "error in"=w387, "AI task in"=w395) -> ("error out"=w376:errorcluster, "Data"=w394:dbl[])  [unwired: 6 in, 1 out]
        n182 = local read "simulate"() -> (w383:bool)
        n183 = Index Array(array=w386, index #1=0 ("index"), index #2=2 ("index")) -> (element #1=w382:bool)  [unwired: 1 out]
        n184 = Index Array(array=w394, index=0) -> (element=w392:dbl)
        n185 = Select(t="10T Sim 2", s=w383, f=w392) -> (s? t:f=w390:dbl)
        n186 = Select(t="<0.1T sim 2", s=w383, f=w382) -> (s? t:f=w380:bool)
        n187 = Less?(x=w390, y=0.1) -> (x < y?=w369:bool)
        n188 = Or(x=w380, y=w369) -> (x .or. y?=w379:bool)
        n189 = Select(t=AR-Auto-Purge."Stop Pump" ("Purge State"), s=w379, f=AR-Auto-Purge."10T Gage") -> (s? t:f=w372:T1)
        n190 = Select(t=w372, s=w373, f=AR-Auto-Purge."End") -> (s? t:f=w370:T1)
        n191 = Merge Errors(w375, w376) -> (w374:errorcluster)
      }
      frame "1000T Gage" {
        # "Auto Purge OFF"
        n192 = call "AR-DI-read.vi"("error in"=w417, "DI task in"=w418) -> ("error out"=w408:errorcluster, "Data"=w416:bool[])  [unwired: 7 in, 1 out]
        n193 = call "AR-AI-read.vi"("number of samples"=10, "error in"=w417, "AI task in"=w425) -> ("error out"=w409:errorcluster, "Data"=w424:dbl[])  [unwired: 6 in, 1 out]
        n194 = local read "simulate"() -> (w413:bool)
        n195 = Index Array(array=w416, index #1=1 ("index"), index #2=2 ("index")) -> (element #1=w402:bool)  [unwired: 1 out]
        n196 = Index Array(array=w424, index=1) -> (element=w422:dbl)
        n197 = Not(x=">750 sim 2") -> (.not. x?=w399:bool)
        n198 = Not(x=w402) -> (.not. x?=w401:bool)
        n199 = Select(t="1000T Sim 2", s=w413, f=w422) -> (s? t:f=w420:dbl)
        n200 = Select(t=w399, s=w413, f=w401) -> (s? t:f=w412:bool)
        n201 = Greater Or Equal?(x=w420, y=7.5) -> (x >= y?=w397:bool)
        n202 = Or(x=w412, y=w397) -> (x .or. y?=w398:bool)
        n203 = case shown="True" w398 {
          frame False {
          }
          frame True {
            n204 = One Button Dialog(message="Now it is safe to open the athmospheric valve to fill the chamber with air. ") -> ()  [unwired: 1 in, 1 out]
          }
        }
        n205 = Select(t=AR-Auto-Purge."End" ("Purge State"), s=w398, f=AR-Auto-Purge."1000T Gage") -> (s? t:f=w405:T1)
        n206 = Select(t=w405, s=w406, f=AR-Auto-Purge."End") -> (s? t:f=w403:T1)
        n207 = Merge Errors(w408, w409) -> (w407:errorcluster)
      }
      frame "End" {
        w431 = T4."Enabled" ("Disabled")
        w433 = FALSE ("Vac SOL")
        w434 = FALSE
        n208 = call "AR-Select-Single-DO.vi"("Action"=AR-DO-Action."Keep DO3") -> ("DO Data"=w438:bool[])  [unwired: 9 in, 1 out]
        n209 = call "AR-DO-write.vi"("error in (no error)"=w436, "Data"=w438, "DO task in"=w437) -> ("error out"=w435:errorcluster)  [unwired: 7 in, 1 out]
        n210 = property on="Pump (DO0)" class="Bool (strict)"(error in=w435, "Value"=w434) -> (error out=w430:errorcluster)  [unwired: 1 in, 1 out]
        n211 = property on="Vac sol (DO1)" class="Bool (strict)"("Value"=w434) -> ()  [unwired: 2 in, 2 out]
        n212 = property on="Gas sol (DO2)" class="Bool (strict)"("Value"=w434) -> ()  [unwired: 2 in, 2 out]
        n213 = local write "Gas SOL"(w433) -> ()
        n214 = local write "Vac SOL"(w433) -> ()
        n215 = local write "O2 pwr"(w433) -> ()
        n216 = property on="Pump (DO0)" class="Bool (strict)"(error in=w430, "DisabledEnum"=w431) -> ()  [unwired: 1 in, 2 out]
        n217 = property on="Vac sol (DO1)" class="Bool (strict)"("DisabledEnum"=w431) -> ()  [unwired: 2 in, 2 out]
        n218 = property on="Gas sol (DO2)" class="Bool (strict)"("DisabledEnum"=w431) -> ()  [unwired: 2 in, 2 out]
        n219 = local write "Auto purge"(FALSE ("Auto purge")) -> ()
        n220 = property on="Auto fill" class="Bool (strict)"("DisabledEnum"=w431) -> ()  [unwired: 2 in, 2 out]
        "Purge Done" <- TRUE ("Fill Done")
      }
    }
    n221 = call "Stop-FGV.vi"("Action (RD)"=enum16{"Init", "WR", "RD"}."RD", "error in"=w300) -> ("error out"=w307:errorcluster, "Out"=w308:bool)  [unwired: 8 in]
    n222 = Compound Arithmetic op=OR(w308, w307) -> (w305:bool)
    "Purge State" <- w302
  }
  n223 = call "Stop-FGV.vi"("Action (RD)"=enum16{"Init", "WR", "RD"}."WR", "error in"=w8, "Action"=TRUE) -> ("error out"=w7:errorcluster)  [unwired: 7 in, 1 out]
  n224 = call "AR-DI-close.vi"("error in (no error)"=w7, "DI task in"=w19) -> ("error out"=w16:errorcluster)  [unwired: 9 in]
  n225 = call "AR-AI-close.vi"("error in (no error)"=w7, "AI task in"=w18) -> ("error out"=w15:errorcluster)  [unwired: 9 in]
  n226 = call "AR-DO-close.vi"("error in (no error)"=w7, "DO task in"=w20) -> ("error out"=w17:errorcluster)  [unwired: 9 in]
  n227 = Merge Errors(w17, w16, w15) -> ()  [unwired: 1 out]
